vi "Draw Speaker Array.vi"(0 "State":T1={"Nspeakers"=13, "actions"=[], "Wspeaker"=13, "hover"={"type"=enum."None", "index"=0}, "locked"=FALSE, "states"=[], "sel speak"=13, "selected"=refnum, "Events"={"Selection change"=refnum}}, 7 "Layout":T6) -> (8 "2D Picture":picture)   [LabVIEW 2020, in "SAC Config.xctl"]
uses:
  SAC Config.xctl
  Layout.ctl
  Item.ctl
  State.vi
  Hover Data.ctl
  Hover Item.ctl
  Speaker State.ctl
  Events.ctl
  Selection changed.ctl
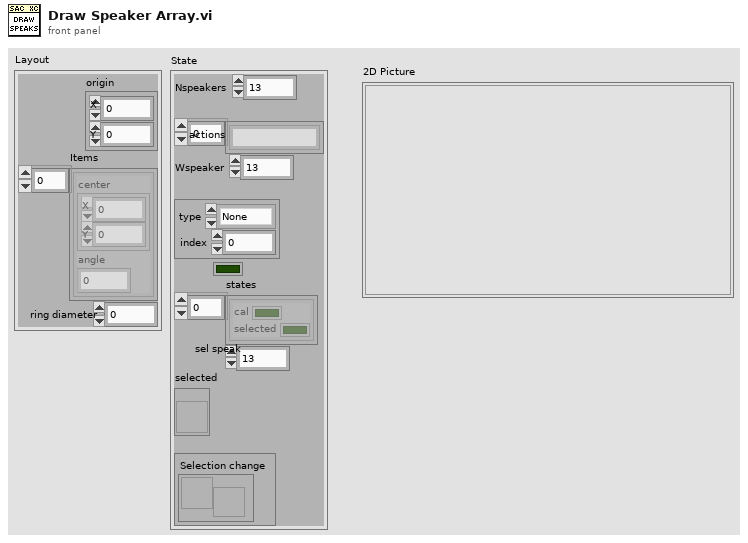
[diagram p1: front panel]
types:
  T1 = typedef "SAC Config.xctl/State.vi" = cluster{"Nspeakers":i32, "actions":string[], "Wspeaker":i32, "hover":T2, "locked":bool, "states":T4[], "sel speak":i32, "selected":refnum<vi>, "Events":T5}
  T2 = typedef "SAC Config.xctl/Hover Data.ctl" = cluster{"type":T3, "index":i32}
  T3 = typedef "SAC Config.xctl/Hover Item.ctl" = enum16{"None", "Speaker"}
  T4 = typedef "SAC Config.xctl/Speaker State.ctl" = cluster{"cal":bool, "selected":bool}
  T5 = typedef "SAC Config.xctl/Events.ctl" = cluster{"Selection change":refnum<user-event>}
  T6 = typedef "SAC Config.xctl/Layout.ctl" = cluster{"origin":cluster{"X":i32, "Y":i32}, "Items":T7[], "ring diameter":i32}
  T7 = typedef "SAC Config.xctl/Item.ctl" = cluster{"center":cluster{"X":i32, "Y":i32}, "angle":dbl}
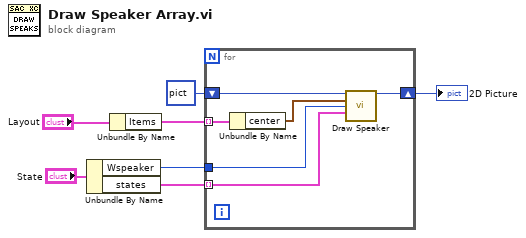
[diagram p0: block diagram]
diagram:
  n1 = Unbundle By Name("State") -> ("Wspeaker"=w3:i32, "states"=w1:T4[])
  n2 = Unbundle By Name("Layout") -> ("Items"=w6:T7[])
  n3 = for {
    shift-right: [w12] -> w5
    shift-left: picture data[5B] ("picture out") -> [w11]
    tunnel: w6 -> [w13] mode=indexing
    tunnel: w3 -> [w9]
    tunnel: w1 -> [w8] mode=indexing
    n4 = Unbundle By Name(w13) -> ("center"=w10:cluster{"X":i32, "Y":i32})
    n5 = call "Draw Speaker.vi"("picture in"=w11, "center"=w10, "width"=w9, "state"=w8) -> ("picture out"=w12:picture)  [unwired: 11 in]
  }
  "2D Picture" <- w5
